vi "connectCommand.vi"(8 "error in (no error)":errorcluster, 11 "MiddlewareSVThisComponent in":refnum<class "MiddlewareSVThisComponent.lvclass">) -> (0 "error out":errorcluster, 3 "MiddlewareSVThisComponent out":refnum<class "MiddlewareSVThisComponent.lvclass">)   [LabVIEW 2015, in "MiddlewareSVThisComponent.lvclass"]
uses:
  MiddlewareSVThisComponent.lvclass
  ComponentTemplateCore/ComponentModel/ComponentModel/Typedefs/CommunicationConfig.ctl
  ComponentTemplateCore/ComponentModel/ComponentModel/Typedefs/SVProcessConfig.ctl
  ComponentTemplateCore/ComponentModel/ComponentModelDT/ConfigurationFileReaderDT/ConfigurationFileReaderDT.lvclass
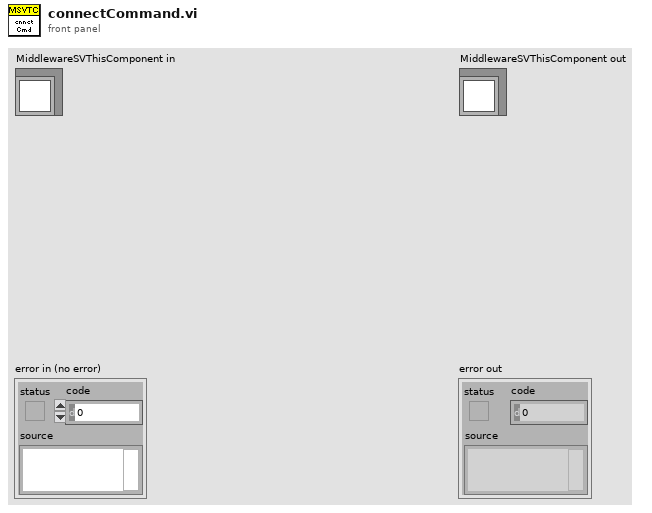
[diagram p1: front panel]
types:
  T1 = typedef "SVProcessConfig.ctl" = cluster{"subDataProcessPrototype":string, "pubDataProcessPrototype":string, "commandProcessPrototype":string, "commandSVName":string}
  T2 = typedef "CommunicationConfig.ctl" = cluster{"hostComputerAddress":string, "ComponentAcronym":string, "InstanceIdentifier":i32}
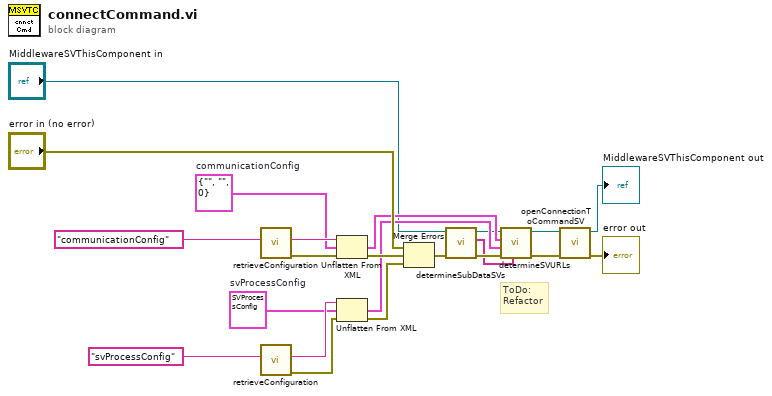
[diagram p0: block diagram]
diagram:
  w15 = T1 {"subDataProcessPrototype"="SubDataSV", "pubDataProcessPrototype"="PubDataSV", "commandProcessPrototype"="CommandSV", "commandSVName"="Command"}  # svProcessConfig
  w19 = T2 {"hostComputerAddress"="", "ComponentAcronym"="", "InstanceIdentifier"=0}  # communicationConfig
  # "ToDo:\nRefactor"
  n1 = call "retrieveConfiguration.vi"("dataName"="communicationConfig") -> ("error out"=w20:errorcluster, "dataValueFromFile"=w21:string)  [unwired: 8 in, 1 out]
  n2 = call "retrieveConfiguration.vi"("dataName"="svProcessConfig") -> ("error out"=w18:errorcluster, "dataValueFromFile"=w17:string)  [unwired: 8 in, 1 out]
  n3 = Unflatten From XML(xml string=w21, type=w19, error in (no error)=w20) -> (value=w6:T2, error out=w14:errorcluster)
  n4 = Unflatten From XML(xml string=w17, type=w15, error in (no error)=w18) -> (value=w7:T1, error out=w13:errorcluster)
  n5 = Merge Errors("error in (no error)", w14, w13) -> (w4:errorcluster)
  n6 = call "determineSubDataSVs.vi"("error in (no error)"=w4, "MiddlewareSVThisComponent in"="MiddlewareSVThisComponent in") -> ("error out"=w3:errorcluster, "svNames"=w1:string[], "MiddlewareSVThisComponent out"=w2:refnum<class "MiddlewareSVThisComponent.lvclass">)  [unwired: 7 in]
  n7 = call-dynamic "determineSVURLs.vi"("SVNames"=w1, "error in (no error)"=w3, "svProcessConfig"=w7, "communicationConfig"=w6, "MiddlewareSV in"=w2) -> ("error out"=w9:errorcluster, "MiddlewareSV out"=w11:refnum<class "MiddlewareSVThisComponent.lvclass">)  [unwired: 5 in]
  n8 = call-dynamic "openConnectionToCommandSV.vi"("error in (no error)"=w9, "MiddlewareSV in"=w11) -> ("error out"=→"error out":errorcluster, "MiddlewareSV out"=→"MiddlewareSVThisComponent out":refnum<class "MiddlewareSVThisComponent.lvclass">)  [unwired: 8 in]
